vi "Read Index.vi"(3 "Index_Pointer)":refnum<class "Index_Pointer.lvclass">) -> (1 "Index Out":i32)   [LabVIEW 2024, in "Index_Pointer.lvclass"]
uses:
  Index_Pointer.lvclass
  Index_Pointer.lvclass/Index_Pointer.ctl
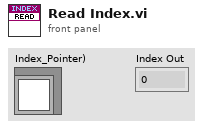
[diagram p1: front panel]
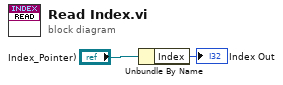
[diagram p0: block diagram]
diagram:
  n1 = Unbundle By Name("Index_Pointer)") -> ("Index"=→"Index Out":i32)
